vi "Create LED Names_LE.vi"(11 "Error In":errorcluster) -> (4 "Names":string[](array[string]), 15 "Error Out":errorcluster)   [LabVIEW 2016, in "TLMB.lvlib"]
uses:
  Projects/TLMB.lvlib
  controls/LEUI_LEDs.ctl
panel:
  in  "LEUI_LEDs_Actual":T1
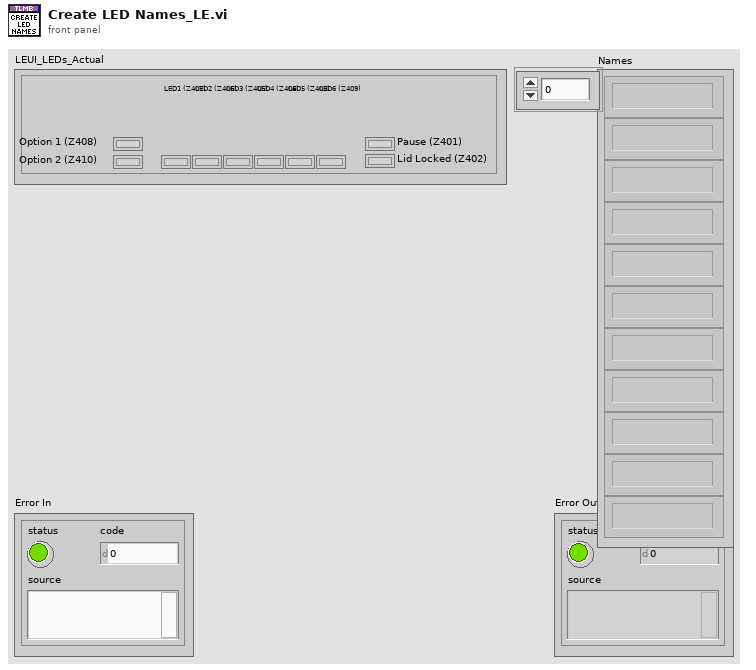
[diagram p1: front panel]
types:
  T1 = typedef "TLMB.lvlib/LEUI_LEDs.ctl" = cluster{"Pause (Z401)":bool, "Lid Locked (Z402)":bool, "LED1 (Z407)":bool, "LED2 (Z406)":bool, "LED3 (Z405)":bool, "LED4 (Z404)":bool, "LED5 (Z403)":bool, "LED6 (Z409)":bool, "Option 1 (Z408)":bool, "Option 2 (Z410)":bool}
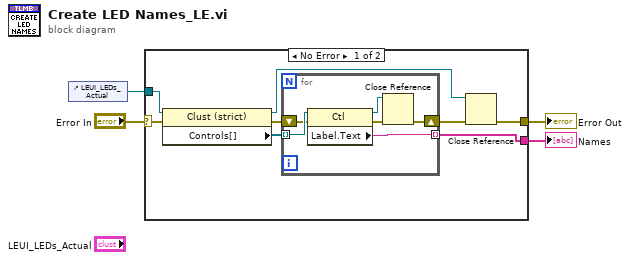
[diagram p0: block diagram]
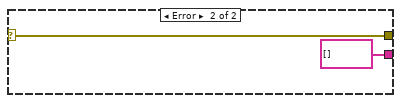
[diagram p2: hidden frame]
diagram:
  n1 = control-ref of="LEUI_LEDs_Actual"() -> (w1:refnum<vi>)
  n2 = case shown="No Error" "Error In" {
    selector: "Error In" -> [w7 w20]
    tunnel: [w8 w20] -> w4
    tunnel: [w6 string[] []] -> w2
    tunnel: w1 -> [w5 _]
    frame No Error {
      n3 = property class="Clust (strict)"(reference=w5, error in=w7) -> (reference out=w9:refnum<vi>, error out=w11:errorcluster, "Controls[]"=w12:refnum<vi>[])
      n4 = for {
        tunnel: w12 -> [w18] mode=indexing
        shift-right: [w14] -> w10
        shift-left: w11 -> [w17]
        tunnel: [w13] -> w6 mode=indexing
        n5 = property class="Ctl"(reference=w18, error in=w17) -> (reference out=w16:refnum<vi>, error out=w15:errorcluster, "Label.Text"=w13:string)
        n6 = Close Reference(reference=w16, error in (no error)=w15) -> (error out=w14:errorcluster)
      }
      n7 = Close Reference(reference=w9, error in (no error)=w10) -> (error out=w8:errorcluster)
    }
    frame Error {
    }
  }
  "Error Out" <- w4
  "Names" <- w2
